vi "Read FTE.vi"(8 "error in":errorcluster, 11 "CoreOOB_Rx in":refnum<class "CIFTemplateCoreOOB_Rx.lvclass">) -> (0 "error out":errorcluster, 2 "FTE":u64, 3 "CoreOOB_Rx out":refnum<class "CIFTemplateCoreOOB_Rx.lvclass">)   [LabVIEW 2021, in "CIFTemplateCoreOOB_Rx.lvclass"]
uses:
  CIFTemplateCoreOOB_Rx.lvclass
  D:/dev/CIF-Core-LabVIEW/src/CIF_Utilities/CifOutOfBand/CIFOutOfBand.lvclass
  CIFUtilities/CifOutOfBand/CIFOutOfBand.lvclass/CIFOutOfBand.ctl
  CIFUtilities/CIFOutOfBand/Accessors/Read Local OOB Data.vi
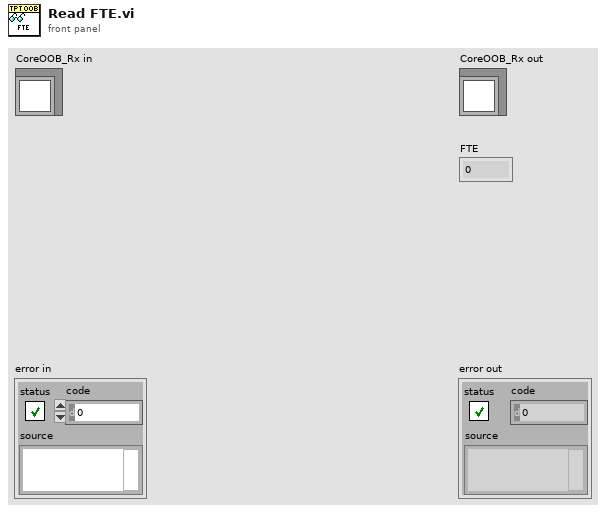
[diagram p1: front panel]
types:
  T1 = typedef "CIFTemplateCoreOOB_Rx.lvclass/Template Payload.ctl" = cluster{"Config Data":variant, "FTE":u64}
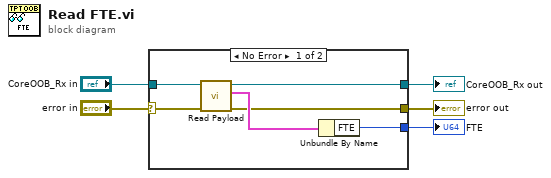
[diagram p0: block diagram]
diagram:
  n1 = case shown="No Error" "error in" {
    selector: "error in" -> [w7 w12]
    tunnel: [w6 w12] -> w4
    tunnel: [w10 w13] -> w2
    tunnel: "CoreOOB_Rx in" -> [w11 w13]
    tunnel: [w8 _] -> w1
    frame No Error {
      n2 = call "Read Payload.vi"("error in"=w7, "CoreOOB_Rx in"=w11) -> ("error out"=w6:errorcluster, "data"=w9:T1, "CoreOOB_Rx out"=w10:refnum<class "CIFTemplateCoreOOB_Rx.lvclass">)  [unwired: 7 in]
      n3 = Unbundle By Name(w9) -> ("FTE"=w8:u64)
    }
    frame Error {
    }
  }
  "error out" <- w4
  "CoreOOB_Rx out" <- w2
  "FTE" <- w1
